vi "CV_sequential.vi"() -> ()   [LabVIEW 2013]
uses:
  InstrControl/Switching/Switching.lvclass
  general_VIs/globals/QC_RunInformation.vi
  InstrControl/InstrControl.lvclass
panel:
  in  "Get all":bool
  in  "Remove Button":bool
  in  "Quit":bool
  in  "Continue":bool
  out "DB Serial Nos.":string[](array[string])
  in  "New Button":bool
  in  "Add Button":bool
  in  "Hardware Configurations":bool
  out "Channel Nos.":string[](array[string])
  # "Sensor QC: sequential CV"
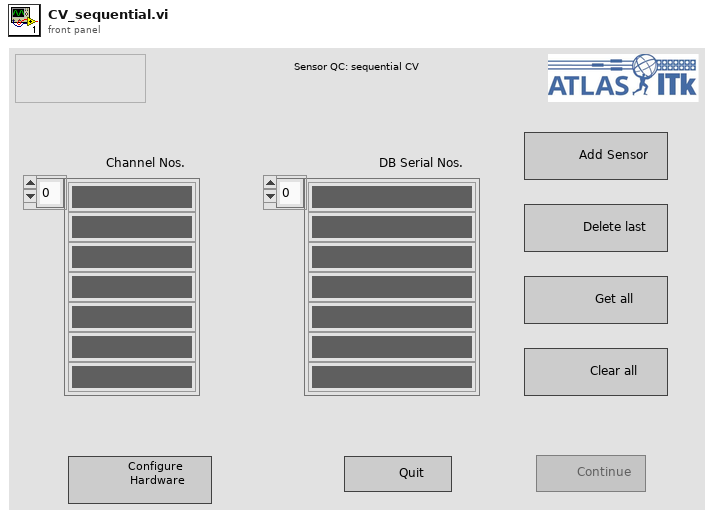
[diagram p1: front panel]
types:
  T1 = enum16{"Supply", "LCR", "Multimeter", "Switching"}
  T2 = cluster{"Institute":string, "Manufacturers":string[], "Devices":string[], "Serialnumbers Lookup DB":string, "Data directory":string, "Backup & screenshot directory":string, "List of known users":string[], "Measurement switch not used":bool, "Measurement Switch":string, "DUT Switch":string, "Rseries IV [MOhm]":string, "Rshunt IV [MOhm]":string, "Rseries CV [MOhm]":string, "DC blocking Cap [µF]":string, "Rseries LCR [MOhm]":string, "Rseries stability [MOhm]":string, "Rshunt stability [MOhm]":string, "Rseries striptest bias [MOhm]":string, "Rseries strip pinhole [MOhm]":string}
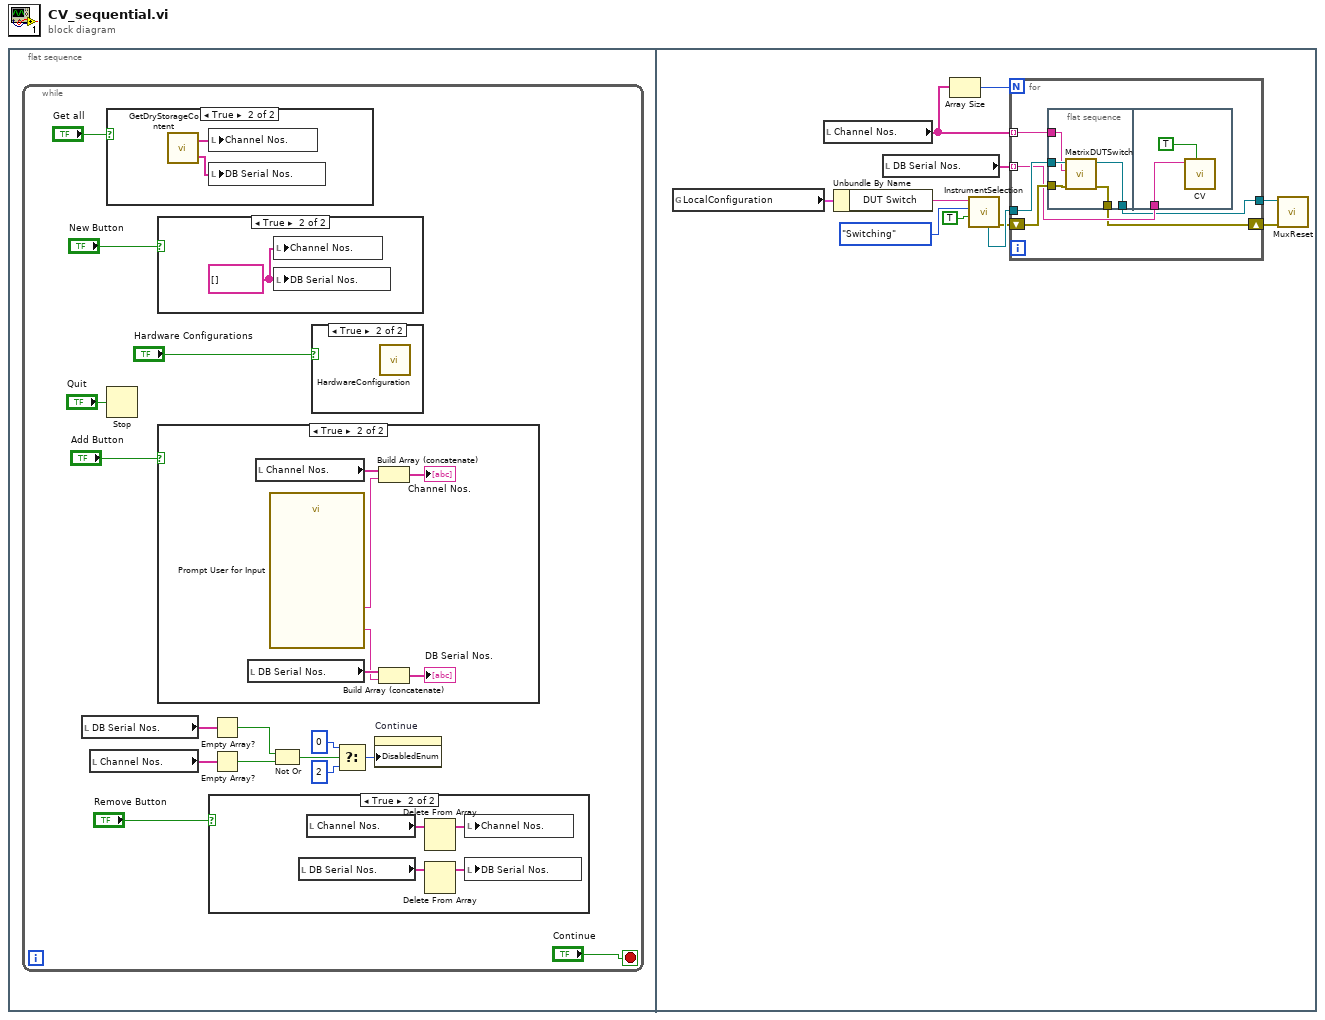
[diagram p0: block diagram]
diagram:
  n1 = flat-sequence {
    frame #0 {
      n2 = while {
        stop <- "Continue" stop-if-true
        n3 = local read "DB Serial Nos."() -> (w11:string[])
        n4 = local read "Channel Nos."() -> (w12:string[])
        n5 = case shown="True" "Get all" {
          frame False {
          }
          frame True {
            n6 = call "GetDryStorageContent.vi"() -> ("DB Serial Nos."=w20:string[], "Channel Nos."=w21:string[])  [unwired: 2 in]
            n7 = local write "Channel Nos."(w21) -> ()
            n8 = local write "DB Serial Nos."(w20) -> ()
          }
        }
        n9 = Stop(stop? (T)="Quit") -> ()
        n10 = case shown="True" "New Button" {
          frame False {
          }
          frame True {
            w22 = string[] [] ("Channel Nos.")
            n11 = local write "Channel Nos."(w22) -> ()
            n12 = local write "DB Serial Nos."(w22) -> ()
          }
        }
        n13 = case shown="True" "Add Button" {
          frame False {
          }
          frame True {
            n14 = local read "DB Serial Nos."() -> (w25:string[])
            n15 = local read "Channel Nos."() -> (w28:string[])
            n16 = call "Prompt User for Input"() -> ("DB serial no."=w24:string, "channel no."=w26:string)  [unwired: 16 in, 2 out]
            n17 = Build Array (concatenate)(w28, w26) -> (→"Channel Nos.":string[])
            n18 = Build Array (concatenate)(w25, w24) -> (→"DB Serial Nos.":string[])
          }
        }
        n19 = case shown="True" "Remove Button" {
          frame False {
          }
          frame True {
            n20 = local read "DB Serial Nos."() -> (w16:string[])
            n21 = local read "Channel Nos."() -> (w17:string[])
            n22 = Delete From Array(array=w17) -> (array with subset deleted=w19:string[])  [unwired: 2 in, 1 out]
            n23 = Delete From Array(array=w16) -> (array with subset deleted=w18:string[])  [unwired: 2 in, 1 out]
            n24 = local write "Channel Nos."(w19) -> ()
            n25 = local write "DB Serial Nos."(w18) -> ()
          }
        }
        n26 = Empty Array?(array=w11) -> (empty?=w10:bool)
        n27 = Empty Array?(array=w12) -> (empty?=w9:bool)
        n28 = Not Or(1:w9, 2:w10) -> (0:w5:bool)
        n29 = case shown="True" "Hardware Configurations" {
          frame False {
          }
          frame True {
            n30 = call "HardwareConfiguration.vi"() -> ()  [unwired: 11 in, 1 out]
          }
        }
        n31 = Select(t=0, s=w5, f=2) -> (s? t:f=w4:i32)
        n32 = property on="Continue" class="Bool"("DisabledEnum"=w4) -> ()  [unwired: 2 in, 2 out]
      }
    }
    frame #1 {
      n33 = global read "QC_RunInformation.vi" "LocalConfiguration"() -> (w39:T2)
      n34 = local read "Channel Nos."() -> (w33:string[])
      n35 = Unbundle By Name(w39) -> ("DUT Switch"=w38:string)
      n36 = local read "DB Serial Nos."() -> (w34:string[])
      n37 = Array Size(array=w33) -> (size(s)=w35:i32)
      n38 = call "InstrumentSelection.vi"("Verify GPIB address"=TRUE, "Instrument type"=T1."Switching", "Instrument name IN"=w38) -> ("error out"=w31:errorcluster, "Switching"=w32:refnum<class "Switching.lvclass">)  [unwired: 3 in, 4 out]
      n39 = for {
        N: w35 -> [_]
        tunnel: w34 -> [w42] mode=indexing
        tunnel: w33 -> [w44] mode=indexing
        tunnel: w32 -> [w45]
        tunnel: [w41] -> w30
        shift-right: [w40] -> w29
        shift-left: w31 -> [w43]
        n40 = flat-sequence {
          tunnel: w45 -> [w50]
          tunnel: w44 -> [w49]
          tunnel: w43 -> [w48]
          tunnel: [w47] -> w41
          tunnel: [w46] -> w40
          tunnel: w42 -> [w51]
          frame #0 {
            n41 = call-dynamic "MatrixDUTSwitch.vi"("error in (no error)"=w48, "Channel #"=w49, "Switching in"=w50) -> ("error out"=w46:errorcluster, "Switching out"=w47:refnum<class "Switching.lvclass">)  [unwired: 7 in]
          }
          frame #1 {
            n42 = call "CV.vi"("Run uninterrupted?"=TRUE, "DB Serial No. IN:"=w51) -> ()  [unwired: 4 in, 1 out]
          }
        }
      }
      n43 = call-dynamic "MuxReset.vi"("error in (no error)"=w29, "Switching in"=w30) -> ()  [unwired: 8 in, 2 out]
    }
  }
